vi "Execute.vi"(8 "error in (no error)":errorcluster, 10 "System In":refnum<class "bt_System.lvclass">, 11 "Node in":refnum<class "Set Double Float.lvclass">) -> (0 "error out":errorcluster, 1 "Status":T1, 2 "System Out":refnum<class "bt_System.lvclass">, 3 "Node out":refnum<class "Set Double Float.lvclass">)   [LabVIEW 2021, in "BT AbsType.lvlib" / "Set Double Float.lvclass"]
uses:
  Set Double Float.lvclass
  C:/Users/Tim/Documents/GitHub/LV_Behaviour_Tree/BT Abstract Type/abs_Type Leaf/abs_Type Leaf.lvclass
  Source/Support/Nodes/abs_Node/Status.ctl
  Source/Support/abs_System/bt_System.lvclass
  <vilib>/TSA/Abstract Data Classes/Abs_Types/Double Float/Abs_Double Float.lvclass
  C:/Program Files (x86)/National Instruments/LabVIEW 2021/vi.lib/TSA/Abstract Data Classes/Abs_Types/Type/Abs_Type.lvclass
  abs_Type Leaf/abs_Type Leaf.lvclass/abs_Type Leaf.ctl
  Set Double Float.lvclass/Set Double Float.ctl
  abs_Type Leaf/Properties/Read Value Class.vi
  Properties/Read Value.vi
  abs_Type Leaf/Properties/Write Value Class.vi
  <vilib>/TSA/Abstract Data Classes/Abs_Types/Type/Abs_Type.lvclass
  abs_Type Leaf/abs_Type Leaf.lvclass
  Source/Support/Nodes/abs_Node/bt_Node.lvclass
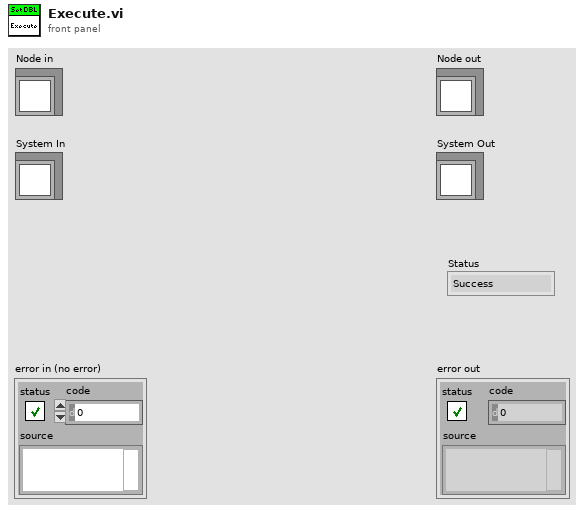
[diagram p1: front panel]
types:
  T1 = typedef "BT.lvlib/bt_Node.lvclass/Status.ctl" = enum16{"Success", "Failure", "Running"}
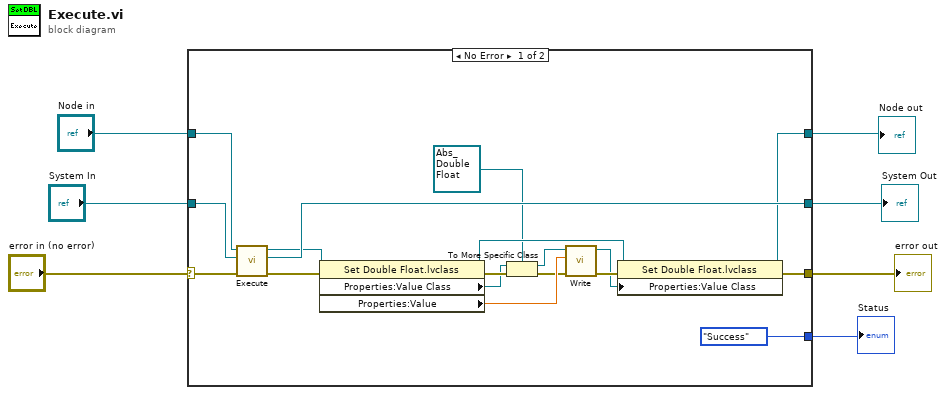
[diagram p0: block diagram]
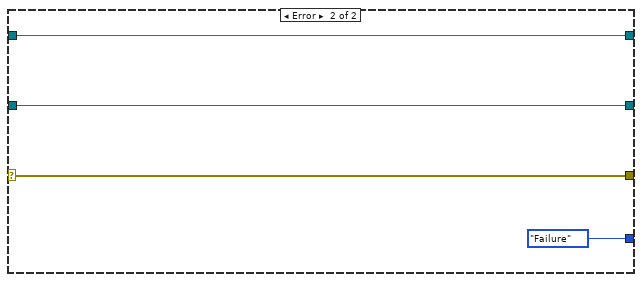
[diagram p2: hidden frame]
diagram:
  n1 = case shown="No Error" "error in (no error)" {
    selector: "error in (no error)" -> [w24 w27]
    tunnel: [w25 w28] -> w4
    tunnel: "System In" -> [w23 w28]
    tunnel: "Node in" -> [w22 w29]
    tunnel: [w18 w27] -> w6
    tunnel: [w17 w29] -> w3
    tunnel: [Status."Success" ("Status") Status."Failure" ("Status")] -> w5
    frame No Error {
      n2 = call-parent "Execute.vi"("error in (no error)"=w24, "System In"=w23, "Node in"=w22) -> ("error out"=w21:errorcluster, "System Out"=w25:refnum<class "bt_System.lvclass">, "Node out"=w20:refnum<class "Set Double Float.lvclass">)  [unwired: 5 in, 1 out]
      n3 = property class="Set Double Float.lvclass"(reference=w20, error in=w21) -> (reference out=w19:refnum<class "Set Double Float.lvclass">, error out=w12:errorcluster, "Properties:Value Class"=w10:refnum<class "Abs_Type.lvclass">, "Properties:Value"=w13:dbl)
      n4 = To More Specific Class(target class=refnum<class "Abs_Double Float.lvclass"> refnum ("Double Float.lvclass_340760 in"), reference=w10, error in=w12) -> (specific class reference=w8:refnum<class "Abs_Double Float.lvclass">, error out=w11:errorcluster)
      n5 = call-dynamic "Write.vi"("error in (no error)"=w11, "Value"=w13, "Double Float.lvclass in"=w8) -> ("error out"=w15:errorcluster, "Double Float.lvclass out"=w14:refnum<class "Abs_Double Float.lvclass">)  [unwired: 7 in]
      n6 = property class="Set Double Float.lvclass"(reference=w19, error in=w15, "Properties:Value Class"=w14) -> (reference out=w17:refnum<class "Set Double Float.lvclass">, error out=w18:errorcluster)
    }
    frame Error {
    }
  }
  "error out" <- w6
  "Node out" <- w3
  "Status" <- w5
  "System Out" <- w4
